vi "DFD Least Pth Norm Design.vi"   [LabVIEW 2017, in "NI_DigFilterLicensed.lvlib"]
doc: "Designs an infinite impulse response (IIR) or finite impulse response (FIR) filter with a frequency response that matches the response you request in terms of the least pth norm algorithm. You can use either the iterative reweighted least square (IRLS) method or the Newton method that this VI provides to design a filter. You must manually select the polymorphic instance you want to use."
uses:
  <vilib>/addons/Digital Filter Design/NI_DigFilterLicensed.lvlib
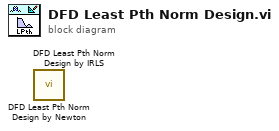
[diagram p0: block diagram]
diagram:
  n1 = call <vilib>:"DFD Least Pth Norm Design by Newton.vi"() -> ()  [unwired: 9 in, 3 out]
  n2 = call <vilib>:"DFD Least Pth Norm Design by IRLS.vi"() -> ()  [unwired: 9 in, 3 out]
